vi "CreateCircle.vi"(10 "Origin":cluster{"x":i16, "y":i16}, 11 "Radius":u16) -> ()   [LabVIEW 2017]
uses:
  Circle/Circle.lvclass
  Point/Point.lvclass
  Graphic/Graphic.lvclass
panel:
  out "Picture":picture
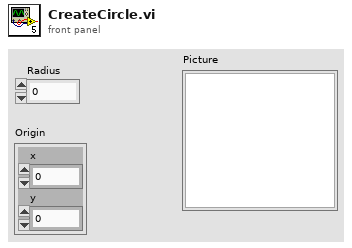
[diagram p1: front panel]
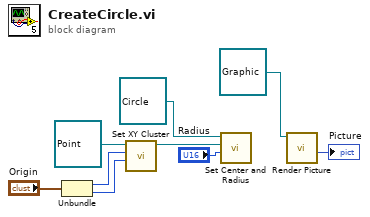
[diagram p0: block diagram]
diagram:
  n1 = Unbundle("Origin") -> ("x"=w6:i16, "y"=w5:i16)
  n2 = call "Set XY Cluster.vi"("Y"=w5, "X"=w6, "Point In"=refnum<class "Point.lvclass"> refnum ("Point.lvclass")) -> ("Point Out"=w4:refnum<class "Point.lvclass">)  [unwired: 8 in]
  n3 = call "Set Center and Radius.vi"("Radius"="Radius", "Point.lvclass"=w4, "Circle in"=refnum<class "Circle.lvclass"> refnum ("Circle.lvclass")) -> ()  [unwired: 8 in, 1 out]
  n4 = call-dynamic "Render Picture.vi"("Graphic In"=refnum<class "Graphic.lvclass"> refnum ("Graphic.lvclass")) -> ("Picture"=→"Picture":picture)  [unwired: 9 in, 1 out]
